vi "Automation Message Loop.vi"(8 "error in (no error)":errorcluster, 9 "Data Queue":refnum<queue>, 10 "Stage Readout Notifier":refnum<notifier>, 11 "Message Queues":T1) -> (0 "error out":errorcluster)   [LabVIEW 2015, in "Automation.lvlib"]
uses:
  Automation.lvlib
  support/Message Queue/All Message Queues.ctl
  support/Message Queue/Message Cluster.ctl
  Automation Configuration.ctl
  Automation State.ctl
  Automation Loop State.ctl
  ZO State.ctl
  ZO Settings.ctl
  Camera/Acquisition Settings.ctl
  Zstack State.ctl
  Zstack Settings.ctl
  Camera/Camera State.ctl
  Camera/Camera Loop State.ctl
  <vilib>/Utility/miscctls.llb/LVMinMaxIncTypeDef.ctl
  Camera/Live View State.ctl
  <vilib>/Utility/error.llb/Error Cluster From Error Code.vi
  <vilib>/ErrorRing/Error Ring.xnode
  support/Message Queue/Message Queue.lvlib
  Camera/Camera.lvlib
  XYZStage/XYZStage.lvlib
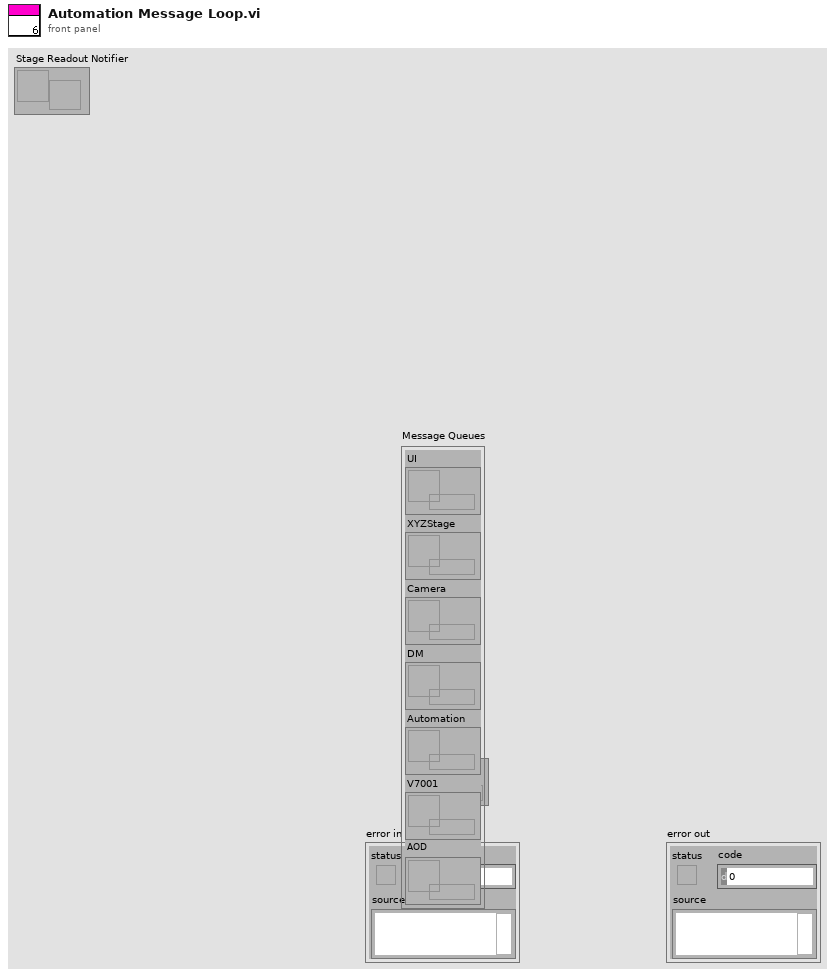
[diagram p1: front panel]
types:
  T1 = typedef "Message Queue.lvlib/All Message Queues.ctl" = cluster{"UI":refnum<queue>, "XYZStage":refnum<queue>, "Camera":refnum<queue>, "DM":refnum<queue>, "Automation":refnum<queue>, "V7001":refnum<queue>, "AOD":refnum<queue>}
  T2 = typedef "Automation.lvlib/Automation State.ctl" = cluster{"Automation State":T3, "Handle out":u32, "ZO State":T4, "Zstack State":T7}
  T3 = typedef "Automation.lvlib/Automation Loop State.ctl" = enum16{"Idle", "Zernike Optimization", "Z Stack"}
  T4 = typedef "Automation.lvlib/ZO State.ctl" = cluster{"ZO Settings":T5, "Zernike Size":i32, "Points per order":i32, "Zernike State":enum16{"Idle", "Waiting for Camera Init.", "Wait for camera frame", "Ready for new mirror config"}, "Zernike Vectors":dbl[][], "Total Frames":i32, "Current Frame":i32}
  T5 = typedef "Automation.lvlib/ZO Settings.ctl" = cluster{"Acquisition Settings":T6, "Shift Amplitude":dbl, "Initial Zernike Vector":dbl[]}
  T6 = typedef "Camera.lvlib/Acquisition Settings.ctl" = cluster{"Save?":bool, "DCIMG Path":path, "Filename":string, "Total Frames":i32, "Sender":enum16{"UI", "Automation"}}
  T7 = typedef "Automation.lvlib/Zstack State.ctl" = cluster{"Zstack Settings":T8, "Zstack State":enum16{"Idle", "Waiting for Camera Init.", "Wait for camera frame", "Ready for new position"}, "Stack Coordinates":dbl[][], "Total Frames":i32, "Current Frame":i32}
  T8 = typedef "Automation.lvlib/Zstack Settings.ctl" = cluster{"Acquisition Settings":T6, "XYZ start":dbl[], "XYZ end":dbl[]}
  T9 = typedef "Automation.lvlib/Automation Configuration.ctl" = cluster{" Index":u32}
  T10 = enum16{"Idle", "Waiting for Camera Init.", "Wait for camera frame", "Ready for new mirror config"}
  T11 = enum16{"Idle", "Waiting for Camera Init.", "Wait for camera frame", "Ready for new position"}
  T12 = typedef "Camera.lvlib/Camera State.ctl" = cluster{"Camera State":T13, "Current Frame":i32, "Handle out":u32, "Camera Details":cluster{"Model":string, "Camera ID":string, "Firmware":string}, "Sub Region":cluster{"H Offset":cluster{"Value":i32, "Limits":T14}, "V Offset":cluster{"Value":i32, "Limits":T14}, "H Size":cluster{"Value":i32, "Limits":T14}, "V Size":cluster{"Value":i32, "Limits":T14}}, "Acquisition Settings":T6, "Live View State":T15}
  T13 = typedef "Camera.lvlib/Camera Loop State.ctl" = enum16{"Idle", "Live View", "Ready", "Acquiring"}
  T14 = typedef "LVMinMaxIncTypeDef.ctl" = cluster{"Minimum":dbl, "Maximum":dbl, "Increment":dbl}
  T15 = typedef "Camera.lvlib/Live View State.ctl" = cluster{"Loop Counter":i32, "Time Of Latest Frame":u32, "Frame Count":u32, "FPS frames":dbl, "FPS Time":u32, "Current FPS":dbl}
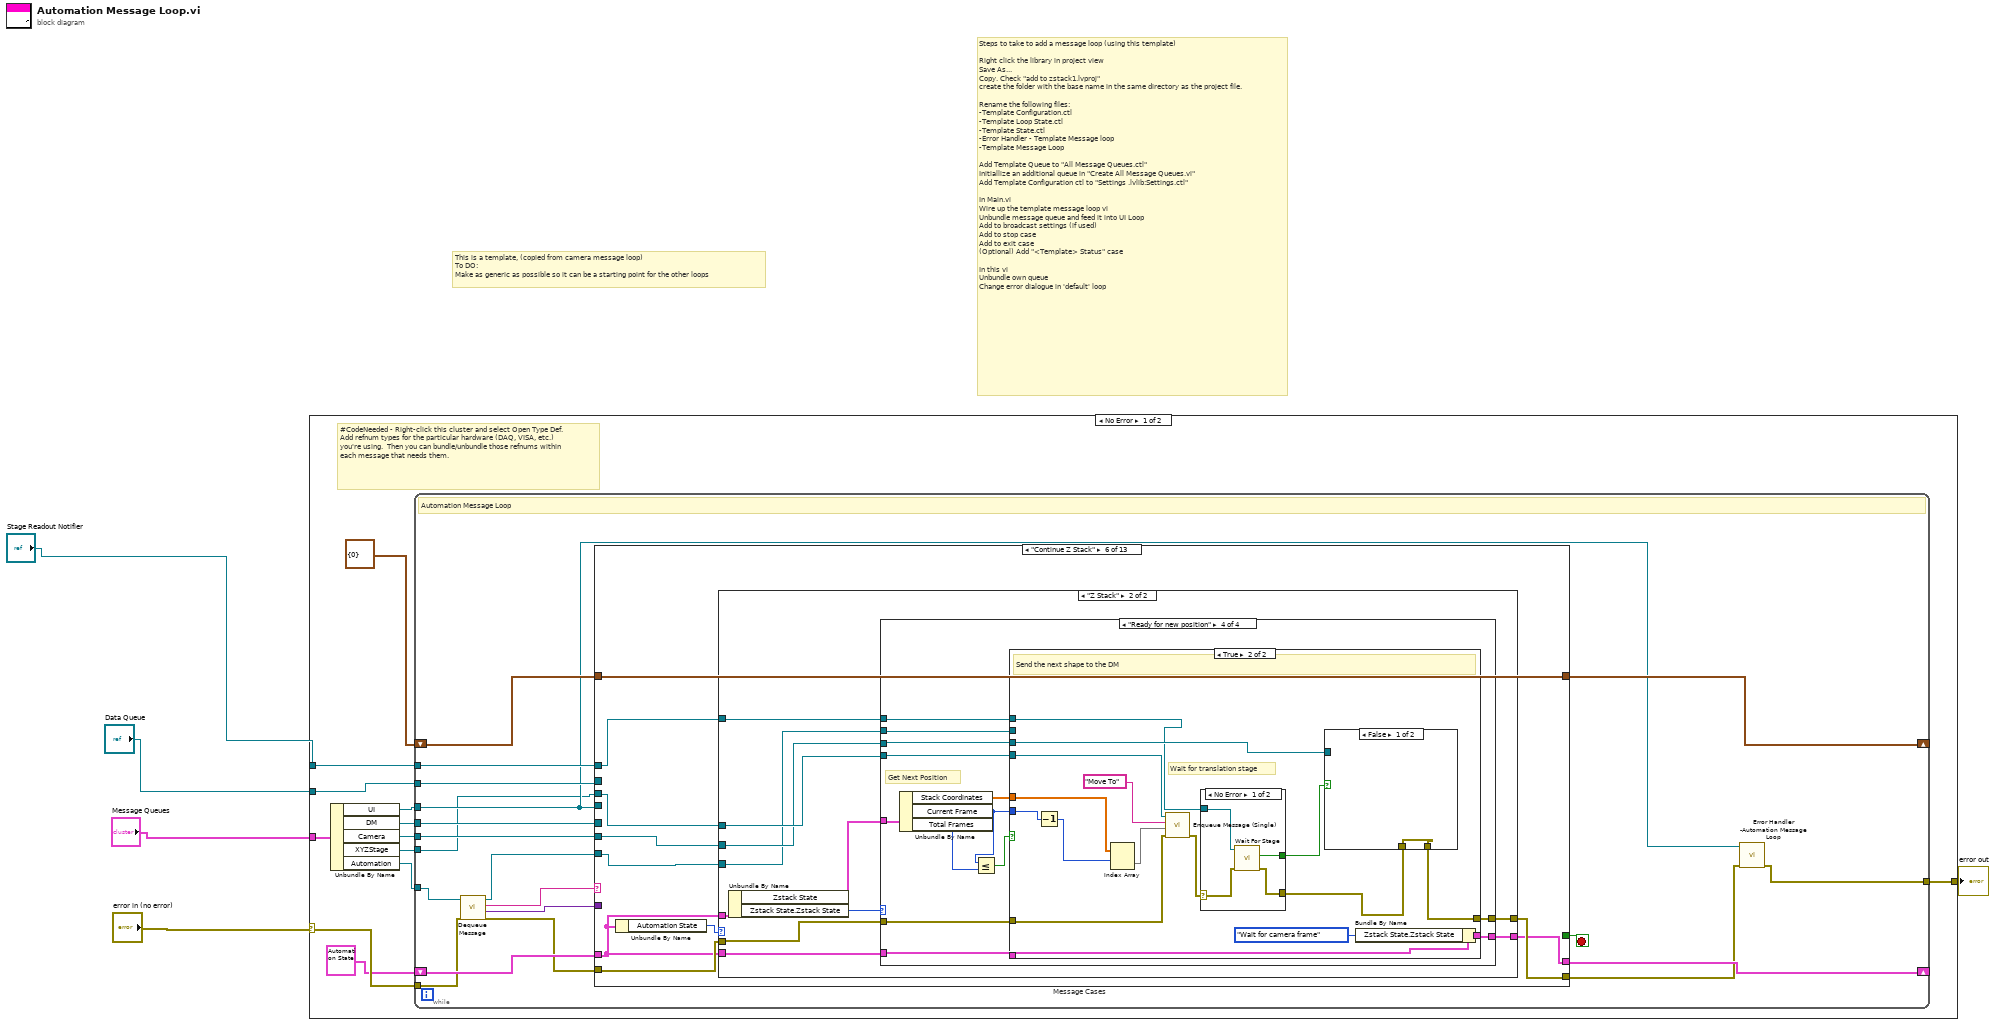
[diagram p0: block diagram]
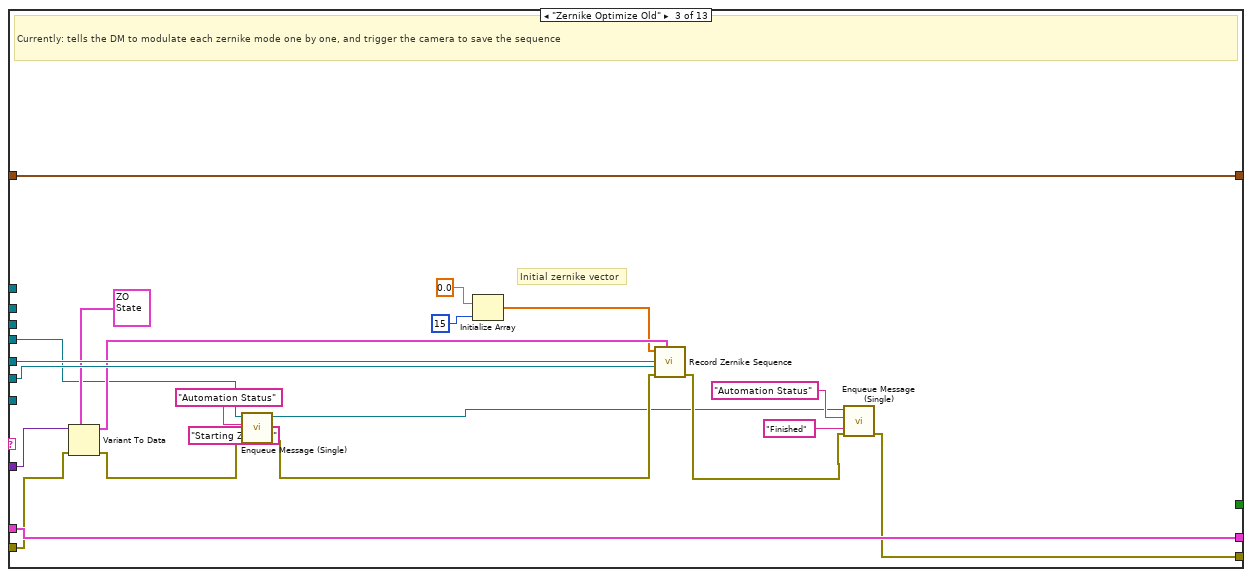
[diagram p4: hidden frame]
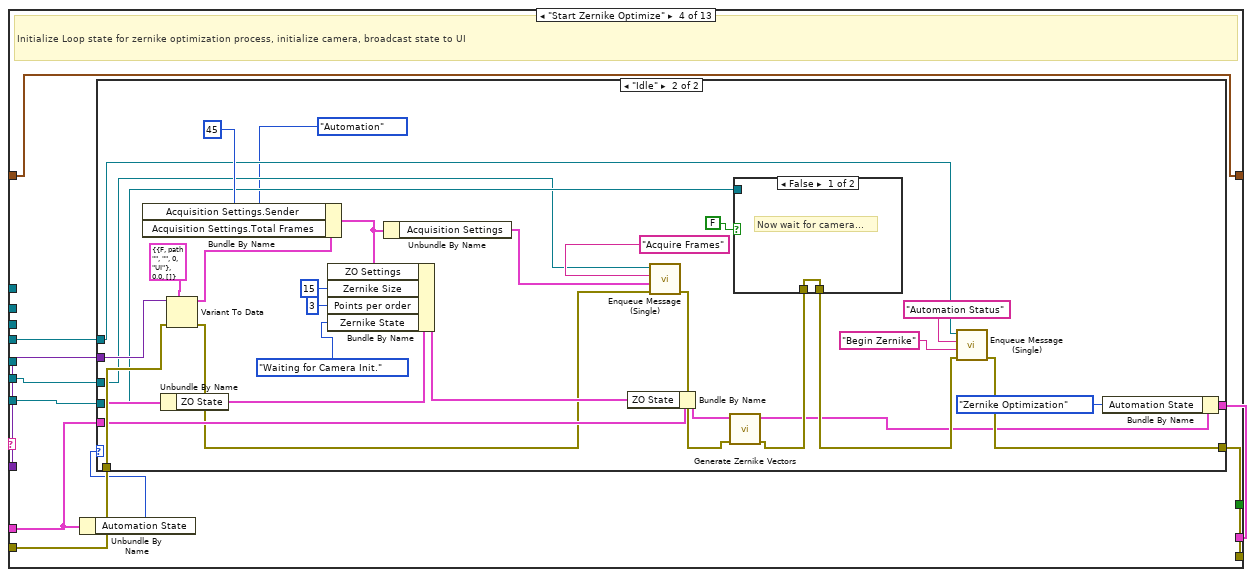
[diagram p5: hidden frame]
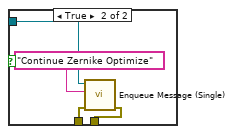
[diagram p7: hidden frame]
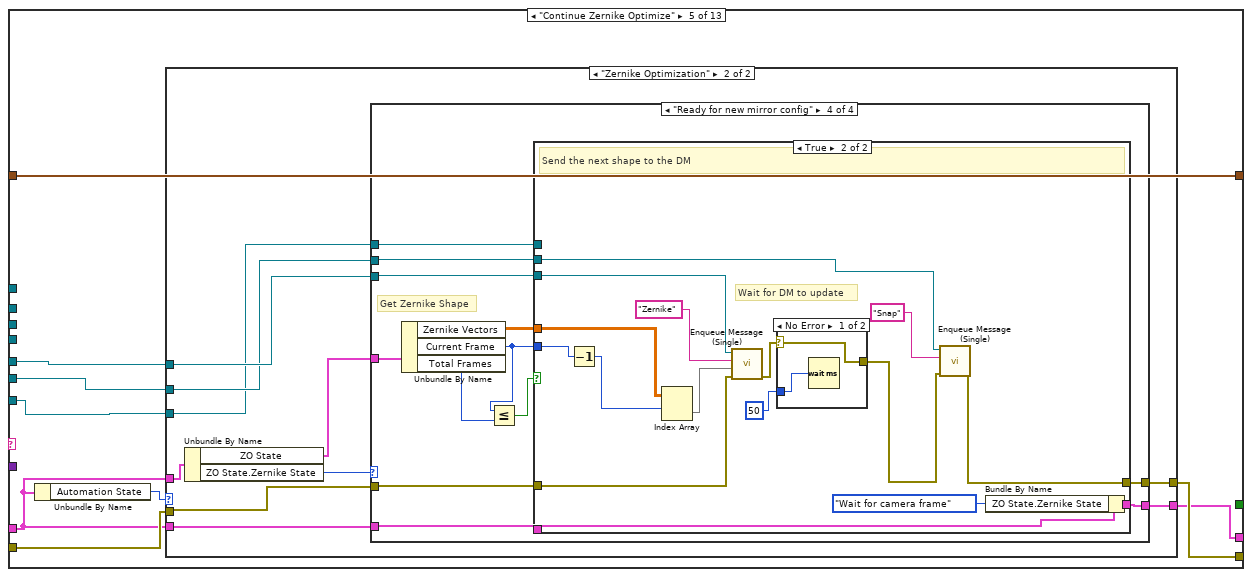
[diagram p8: hidden frame]
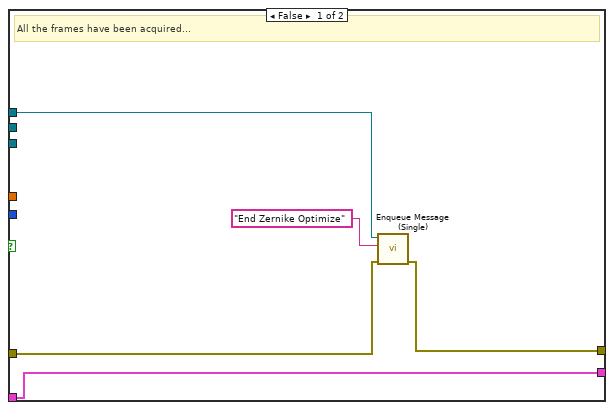
[diagram p13: hidden frame]
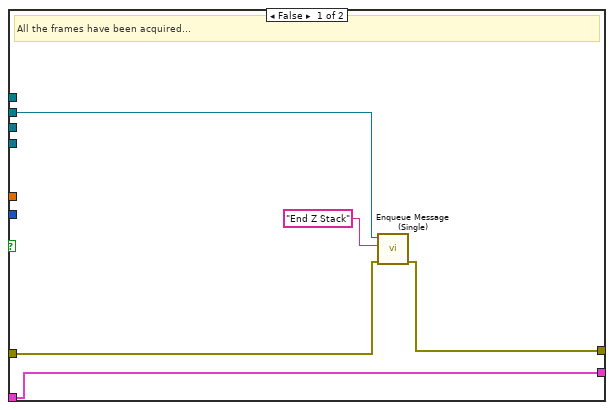
[diagram p19: hidden frame]
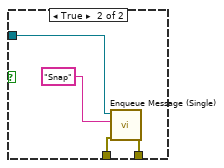
[diagram p20: hidden frame]
diagram:
  # "Steps to take to add a message loop (using this template)\n\nRight click the library in project view\nSave As...\nCopy. Check \"add to zstack1.lvproj\"\ncreate the folder with the base name in the same directory as the project file.\n\nRename the following files:\n-Template Configuration.ctl\n-Template Loop State.ctl\n-Template State.ctl\n-Error Handler - Template Message loop\n-Template Message Loop\n\nAdd Template Queue to \"All Message Queues.ctl\"\nInitiallize an additional queue in \"Create All Message Queues.vi\"\nAdd Template Configuration ctl to \"Settings .lvlib:Settings.ctl\"\n\nIn Main.vi\nWire up the template message loop vi\nUnbundle message queue and feed it into UI Loop\nAdd to broadcast settings (if used)\nAdd to stop case\nAdd to exit case\n(Optional) Add \"<Template> Status\" case\n\nIn this vi\nUnbundle own queue\nChange error dialogue in 'default' loop"
  # "This is a template, (copied from camera message loop)\nTo DO:\nMake as generic as possible so it can be a starting point for the other loops"
  n1 = case shown="No Error" "error in (no error)" {
    selector: "error in (no error)" -> [w15 w469]
    tunnel: "Message Queues" -> [w17 _]
    tunnel: [w16 w469] -> w5
    tunnel: "Stage Readout Notifier" -> [w14 _]
    tunnel: "Data Queue" -> [w13 _]
    frame No Error {
      # "#CodeNeeded - Right-click this cluster and select Open Type Def.  Add refnum types for the particular hardware (DAQ, VISA, etc.) you're using.  Then you can bundle/unbundle those refnums within each message that needs them."
      n2 = Unbundle By Name(w17) -> ("UI"=w10:refnum<queue>, "DM"=w8:refnum<queue>, "Camera"=w7:refnum<queue>, "XYZStage"=w6:refnum<queue>, "Automation"=w9:refnum<queue>)
      n3 = while {
        tunnel: w9 -> [w29]
        shift-right: [w35] -> _
        shift-left: T9 {" Index"=0} ("Hardware Configuration") -> [w36]
        tunnel: w10 -> [w21]
        tunnel: w14 -> [w33]
        tunnel: w13 -> [w32]
        shift-right: [w30] -> _
        shift-left: T2 {"Automation State"=enum."Idle", "Handle out"=0, "ZO State"={"ZO Settings"={"Acquisition Settings"={"Save?"=FALSE, "DCIMG Path"=path "", "Filename"="", "Total Frames"=0, "Sender"=enum."UI"}, "Shift Amplitude"=0.0, "Initial Zernike Vector"=[]}, "Zernike Size"=15, "Points per order"=15, "Zernike State"=enum."Idle", "Zernike Vectors"=[], "Total Frames"=15, "Current Frame"=15}, "Zstack State"={"Zstack Settings"={"Acquisition Settings"={"Save?"=FALSE, "DCIMG Path"=path "", "Filename"="", "Total Frames"=0, "Sender"=enum."UI"}, "XYZ start"=[], "XYZ end"=[]}, "Zstack State"=enum."Idle", "Stack Coordinates"=[], "Total Frames"=15, "Current Frame"=15}} ("Cluster") -> [w31]
        tunnel: w15 -> [w28]
        tunnel: [w23] -> w16
        tunnel: w8 -> [w20]
        tunnel: w7 -> [w19]
        tunnel: w6 -> [w18]
        stop <- w34 stop-if-true
        # "Automation Message Loop"
        n4 = call "Dequeue Message.vi"("error in (no error)"=w28, "Message Queue"=w29) -> ("error out"=w24:errorcluster, "Message Data"=w25:variant, "Message"=w26:string, "dup Message Queue"=w27:refnum<queue>)  [unwired: 6 in]
        n5 = case "Message Cases" shown="\"Continue Z Stack\"" w26 {
          selector: w26 -> [_ _ _ _ _ _ _ _ _ _ _ _ w458]
          tunnel: w27 -> [_ _ _ w68 w111 w176 w255 w285 w306 w331 w448 _ _]
          tunnel: w24 -> [w39 w42 w58 w71 w116 w181 w252 w290 w311 w334 w450 w457 _]
          tunnel: [w39 w42 w44 w70 w115 w180 w251 w289 w310 w329 w452 w455 w459] -> w22
          tunnel: w36 -> [w37 w41 w63 w73 w119 w183 w257 w293 w314 w337 w451 w456 w461]
          tunnel: [w37 w41 w63 w73 w119 w183 w257 w293 w314 w337 w451 w456 w461] -> w35
          tunnel: [_ _ _ _ _ _ _ _ _ _ TRUE _ _] -> w34
          tunnel: w25 -> [_ _ w59 w72 _ _ w248 _ _ w335 _ _ _]
          tunnel: w21 -> [_ _ w51 w69 _ _ w256 w284 w305 _ _ _ _]
          tunnel: w33 -> [_ _ _ _ _ w174 _ _ _ _ _ _ _]
          tunnel: w32 -> [_ _ _ _ _ _ _ _ _ _ _ _ _]
          tunnel: w31 -> [w38 w40 w62 w65 w113 w178 w250 w287 w308 w327 w447 w454 w460]
          tunnel: [w38 w40 w62 w66 w112 w177 w249 w286 w307 w326 w447 w454 w460] -> w30
          tunnel: w20 -> [_ _ w61 _ w117 _ _ w291 w312 _ _ _ _]
          tunnel: w19 -> [_ _ w60 w67 w114 w179 w254 w288 w309 _ _ _ _]
          tunnel: w18 -> [_ _ _ _ _ w175 _ _ _ _ _ _ _]
          frame "Initialize" {
            # "Initialize  - Initialize is currently a no-op.  The hardware initialization takes place in the 'Start' message."
          }
          frame "Stop" {
          }
          frame "Zernike Optimize Old" {
            # "Initial zernike vector"
            # "Currently: tells the DM to modulate each zernike mode one by one, and trigger the camera to save the sequence"
            n6 = Variant To Data(error in=w58, type=T4 {"ZO Settings"={"Acquisition Settings"={"Save?"=FALSE, "DCIMG Path"=path "E:/test2", "Filename"="zernike", "Total Frames"=0, "Sender"=enum."Automation"}, "Shift Amplitude"=0.0, "Initial Zernike Vector"=[]}, "Zernike Size"=15, "Points per order"=15, "Zernike State"=enum."Idle", "Zernike Vectors"=[], "Total Frames"=0, "Current Frame"=15} ("Zernike Optimize Settings"), Variant=w59) -> (data=w56:T4, error out=w50:errorcluster)
            n7 = call "Enqueue Message (Single).vi"("error in (no error)"=w50, "Message Data"="Starting Zernike" ("Message"), "Message"="Automation Status", "Message Queue"=w51) -> ("error out"=w49:errorcluster, "dup Message Queue"=w43:refnum<queue>)  [unwired: 6 in]
            n8 = Initialize Array(0.0 ("element"), 15 ("dimension size")) -> (w55:dbl[])
            n9 = call "Record Zernike Sequence.vi"("Zernike Optimize Settings"=w56, "error in"=w49, "Camera"=w60, "DM"=w61, "Z_0"=w55) -> ("error out"=w45:errorcluster)  [unwired: 6 in]
            n10 = call "Enqueue Message (Single).vi"("error in (no error)"=w45, "Message Data"="Finished" ("Message"), "Message"="Automation Status", "Message Queue"=w43) -> ("error out"=w44:errorcluster)  [unwired: 6 in, 1 out]
          }
          frame "Start Zernike Optimize" {
            # "Initialize Loop state for zernike optimization process, initialize camera, broadcast state to UI"
            n11 = Unbundle By Name(w65) -> ("Automation State"=w64:T3)
            n12 = case shown="\"Idle\"" w64 {
              tunnel: w72 -> [_ w105]
              tunnel: w71 -> [w74 w104]
              tunnel: w65 -> [w75 w103]
              tunnel: [w74 w96] -> w70
              tunnel: w69 -> [_ w95]
              tunnel: w68 -> [_ w94]
              tunnel: w67 -> [_ w91]
              tunnel: [w75 w77] -> w66
              frame Default {
                # "Doing something else!... don't start zernike optimize"
              }
              frame "Idle" {
                n13 = Unbundle By Name(w103) -> ("ZO State"=w99:T4)
                n14 = Variant To Data(error in=w104, type=T5 {"Acquisition Settings"={"Save?"=FALSE, "DCIMG Path"=path "", "Filename"="", "Total Frames"=0, "Sender"=enum."UI"}, "Shift Amplitude"=0.0, "Initial Zernike Vector"=[]} ("ZO Settings"), Variant=w105) -> (data=w100:T5, error out=w88:errorcluster)
                n15 = Bundle By Name(cluster=w100, "Acquisition Settings.Sender"=enum16{"UI", "Automation"}."Automation", "Acquisition Settings.Total Frames"=45) -> (w90:T5)
                n16 = Bundle By Name(cluster=w99, "ZO Settings"=w90, "Zernike Size"=15, "Points per order"=3, "Zernike State"=T10."Waiting for Camera Init.") -> (w98:T4)
                n17 = Unbundle By Name(w90) -> ("Acquisition Settings"=w89:T6)
                n18 = Bundle By Name(cluster=w103, "ZO State"=w98) -> (w82:T2)
                n19 = call "Enqueue Message (Single).vi"("error in (no error)"=w88, "Message Data"=w89, "Message"="Acquire Frames", "Message Queue"=w91) -> ("error out"=w83:errorcluster)  [unwired: 6 in, 1 out]
                n20 = call "Generate Zernike Vectors.vi"("error in (no error)"=w83, "Automation State in"=w82) -> ("error out"=w84:errorcluster, "Automation State Out"=w78:T2)  [unwired: 6 in]
                n21 = case shown="False" FALSE {
                  tunnel: w94 -> [_ w109]
                  tunnel: [w106 w108] -> w93
                  tunnel: w84 -> [w106 w107]
                  frame False {
                    # "Now wait for camera..."
                  }
                  frame True {
                    n22 = call "Enqueue Message (Single).vi"("error in (no error)"=w107, "Message"="Continue Zernike Optimize", "Message Queue"=w109) -> ("error out"=w108:errorcluster)  [unwired: 7 in, 1 out]
                  }
                }
                n23 = call "Enqueue Message (Single).vi"("error in (no error)"=w93, "Message Data"="Begin Zernike" ("Message"), "Message"="Automation Status", "Message Queue"=w95) -> ("error out"=w96:errorcluster)  [unwired: 6 in, 1 out]
                n24 = Bundle By Name(cluster=w78, "Automation State"=Automation_Loop_State."Zernike Optimization") -> (w77:T2)
              }
            }
          }
          frame "Continue Zernike Optimize" {
            n25 = Unbundle By Name(w113) -> ("Automation State"=w118:T3)
            n26 = case shown="\"Zernike Optimization\"" w118 {
              tunnel: w113 -> [_ w131]
              tunnel: w117 -> [_ w128]
              tunnel: w116 -> [w120 w127]
              tunnel: [w120 w126] -> w115
              tunnel: w114 -> [_ w125]
              tunnel: w113 -> [w121 w124]
              tunnel: [w121 w123] -> w112
              tunnel: w111 -> [_ w122]
              frame "Idle", Default {
              }
              frame "Zernike Optimization" {
                n27 = Unbundle By Name(w131) -> ("ZO State"=w129:T4, "ZO State.Zernike State"=w130:T10)
                n28 = case shown="\"Ready for new mirror config\"" w130 {
                  tunnel: w129 -> [_ _ _ w149]
                  tunnel: w128 -> [_ _ _ w147]
                  tunnel: w127 -> [w132 w134 w136 w146]
                  tunnel: [w132 w134 w136 w144] -> w126
                  tunnel: w125 -> [_ _ _ w145]
                  tunnel: w124 -> [w133 w135 w137 w142]
                  tunnel: [w133 w135 w137 w143] -> w123
                  tunnel: w122 -> [_ _ _ w138]
                  frame "Idle", Default {
                  }
                  frame "Waiting for Camera Init." {
                  }
                  frame "Wait for camera frame" {
                  }
                  frame "Ready for new mirror config" {
                    # "Get Zernike Shape"
                    n29 = Unbundle By Name(w149) -> ("Zernike Vectors"=w148:dbl[][], "Current Frame"=w141:i32, "Total Frames"=w140:i32)
                    n30 = Less Or Equal?(x=w141, y=w140) -> (x <= y?=w139:bool)
                    n31 = case shown="True" w139 {
                      tunnel: w148 -> [_ w170]
                      tunnel: w147 -> [_ w165]
                      tunnel: w146 -> [w153 w164]
                      tunnel: w145 -> [_ w163]
                      tunnel: [w152 w160] -> w144
                      tunnel: [w151 w159] -> w143
                      tunnel: w142 -> [w151 w158]
                      tunnel: w141 -> [_ w156]
                      tunnel: w138 -> [w150 _]
                      frame False {
                        # "All the frames have been acquired..."
                        n32 = call "Enqueue Message (Single).vi"("error in (no error)"=w153, "Message"="End Zernike Optimize", "Message Queue"=w150) -> ("error out"=w152:errorcluster)  [unwired: 7 in, 1 out]
                      }
                      frame True {
                        # "Wait for DM to update"
                        # "Send the next shape to the DM"
                        n33 = Decrement(x=w156) -> (x-1=w155:i32)
                        n34 = Index Array(array=w170, index (row)=w155) -> (element=w166:dbl[])  [unwired: 1 in]
                        n35 = call "Enqueue Message (Single).vi"("error in (no error)"=w164, "Message Data"=w166, "Message"="Zernike", "Message Queue"=w165) -> ("error out"=w168:errorcluster)  [unwired: 6 in, 1 out]
                        n36 = case shown="No Error" w168 {
                          selector: w168 -> [w171 w173]
                          tunnel: u32 50 ("milliseconds to wait") -> [w172 _]
                          tunnel: [w171 w173] -> w161
                          frame No Error {
                            n37 = Wait (ms)(milliseconds to wait=w172) -> ()  [unwired: 1 out]
                          }
                          frame Error {
                          }
                        }
                        n38 = call "Enqueue Message (Single).vi"("error in (no error)"=w161, "Message"="Snap", "Message Queue"=w163) -> ("error out"=w160:errorcluster)  [unwired: 7 in, 1 out]
                        n39 = Bundle By Name(cluster=w158, "ZO State.Zernike State"=T10."Wait for camera frame") -> (w159:T2)
                      }
                    }
                  }
                }
              }
            }
          }
          frame "Continue Z Stack" {
            n40 = Unbundle By Name(w178) -> ("Automation State"=w182:T3)
            n41 = case shown="\"Z Stack\"" w182 {
              tunnel: w178 -> [_ w196]
              tunnel: w175 -> [_ w193]
              tunnel: w181 -> [w184 w192]
              tunnel: [w184 w191] -> w180
              tunnel: w179 -> [_ w190]
              tunnel: w178 -> [w185 w189]
              tunnel: [w185 w188] -> w177
              tunnel: w176 -> [_ w187]
              tunnel: w174 -> [_ w186]
              frame "Idle", Default {
              }
              frame "Z Stack" {
                n42 = Unbundle By Name(w196) -> ("Zstack State"=w194:T7, "Zstack State.Zstack State"=w195:T11)
                n43 = case shown="\"Ready for new position\"" w195 {
                  tunnel: w194 -> [_ _ _ w215]
                  tunnel: w193 -> [_ _ _ w213]
                  tunnel: w192 -> [w197 w199 w201 w212]
                  tunnel: [w197 w199 w201 w210] -> w191
                  tunnel: w190 -> [_ _ _ w211]
                  tunnel: w189 -> [w198 w200 w202 w208]
                  tunnel: [w198 w200 w202 w209] -> w188
                  tunnel: w187 -> [_ _ _ w204]
                  tunnel: w186 -> [_ _ _ w203]
                  frame "Idle", Default {
                  }
                  frame "Waiting for Camera Init." {
                  }
                  frame "Wait for camera frame" {
                  }
                  frame "Ready for new position" {
                    # "Get Next Position"
                    n44 = Unbundle By Name(w215) -> ("Stack Coordinates"=w214:dbl[][], "Current Frame"=w207:i32, "Total Frames"=w206:i32)
                    n45 = Less Or Equal?(x=w207, y=w206) -> (x <= y?=w205:bool)
                    n46 = case shown="True" w205 {
                      tunnel: w214 -> [_ w236]
                      tunnel: w213 -> [_ w232]
                      tunnel: w212 -> [w219 w231]
                      tunnel: w211 -> [_ w230]
                      tunnel: [w218 w228] -> w210
                      tunnel: [w217 w227] -> w209
                      tunnel: w208 -> [w217 w226]
                      tunnel: w207 -> [_ w225]
                      tunnel: w204 -> [w216 _]
                      tunnel: w203 -> [_ w221]
                      frame False {
                        # "All the frames have been acquired..."
                        n47 = call "Enqueue Message (Single).vi"("error in (no error)"=w219, "Message"="End Z Stack", "Message Queue"=w216) -> ("error out"=w218:errorcluster)  [unwired: 7 in, 1 out]
                      }
                      frame True {
                        # "Wait for translation stage"
                        # "Send the next shape to the DM"
                        n48 = Decrement(x=w225) -> (x-1=w224:i32)
                        n49 = Index Array(array=w236, index (row)=w224) -> (element=w233:dbl[])  [unwired: 1 in]
                        n50 = call "Enqueue Message (Single).vi"("error in (no error)"=w231, "Message Data"=w233, "Message"="Move To", "Message Queue"=w232) -> ("error out"=w234:errorcluster)  [unwired: 6 in, 1 out]
                        n51 = case shown="No Error" w234 {
                          selector: w234 -> [w245 w247]
                          tunnel: [w244 w247] -> w229
                          tunnel: [w243 FALSE ("In Position")] -> w222
                          tunnel: w221 -> [w242 _]
                          frame No Error {
                            n52 = call "Wait For Stage.vi"("error in (no error)"=w245, "Stage Readout Notifier"=w242) -> ("error out"=w244:errorcluster, "In Position"=w243:bool)  [unwired: 8 in]
                          }
                          frame Error {
                          }
                        }
                        n53 = case shown="False" w222 {
                          tunnel: w230 -> [_ w241]
                          tunnel: w229 -> [w237 w239]
                          tunnel: [w237 w238] -> w228
                          frame False {
                          }
                          frame True {
                            n54 = call "Enqueue Message (Single).vi"("error in (no error)"=w239, "Message"="Snap", "Message Queue"=w241) -> ("error out"=w238:errorcluster)  [unwired: 7 in, 1 out]
                          }
                        }
                        n55 = Bundle By Name(cluster=w226, "Zstack State.Zstack State"=T11."Wait for camera frame") -> (w227:T2)
                      }
                    }
                  }
                }
              }
            }
          }
          frame "Start Z Stack" {
            n56 = Unbundle By Name(w250) -> ("Automation State"=w253:T3)
            n57 = case shown="Default" w253 {
              tunnel: w248 -> [_ w278]
              tunnel: w252 -> [w258 w277]
              tunnel: w250 -> [w259 w265]
              tunnel: [w258 w275] -> w251
              tunnel: w256 -> [_ w274]
              tunnel: w255 -> [_ w273]
              tunnel: w254 -> [_ w270]
              tunnel: [w259 w261] -> w249
              frame Default {
                # "Doing something else!... don't start zernike optimize"
              }
              frame "Idle" {
                # "initialize camera"
                n58 = Variant To Data(error in=w277, type=T8 {"Acquisition Settings"={"Save?"=FALSE, "DCIMG Path"=path "", "Filename"="", "Total Frames"=0, "Sender"=enum."UI"}, "XYZ start"=[], "XYZ end"=[]} ("Zstack Settings"), Variant=w278) -> (data=w264:T8, error out=w263:errorcluster)
                n59 = call "Initialize Z Stack.vi"("error in (no error)"=w263, "Zstack Settings in"=w264, "Automation State in"=w265) -> ("error out"=w262:errorcluster, "Automation State Out"=w261:T2)  [unwired: 5 in]
                n60 = Unbundle By Name(w261) -> ("Zstack State.Zstack Settings.Acquisition Settings"=w260:T6)
                n61 = call "Enqueue Message (Single).vi"("error in (no error)"=w262, "Message Data"=w260, "Message"="Acquire Frames", "Message Queue"=w270) -> ("error out"=w266:errorcluster)  [unwired: 6 in, 1 out]
                n62 = case shown="False" FALSE {
                  tunnel: w273 -> [_ w282]
                  tunnel: [w279 w281] -> w272
                  tunnel: w266 -> [w279 w280]
                  frame False {
                    # "Now wait for camera..."
                  }
                  frame True {
                    n63 = call "Enqueue Message (Single).vi"("error in (no error)"=w280, "Message"="Continue Zernike Optimize", "Message Queue"=w282) -> ("error out"=w281:errorcluster)  [unwired: 7 in, 1 out]
                  }
                }
                n64 = call "Enqueue Message (Single).vi"("error in (no error)"=w272, "Message Data"="Begin Z Stack" ("Message"), "Message"="Automation Status", "Message Queue"=w274) -> ("error out"=w275:errorcluster)  [unwired: 6 in, 1 out]
              }
            }
          }
          frame "End Zernike Optimize" {
            # "Clear settings and set loop state to idle..."
            n65 = Unbundle By Name(w287) -> ("Automation State"=w292:T3)
            n66 = case shown="\"Zernike Optimization\"" w292 {
              tunnel: w287 -> [_ _]
              tunnel: w291 -> [_ _]
              tunnel: w290 -> [w294 w297]
              tunnel: [w294 w296] -> w289
              tunnel: w288 -> [_ _]
              tunnel: w287 -> [w295 w301]
              tunnel: [w295 w300] -> w286
              tunnel: w285 -> [_ _]
              tunnel: w284 -> [_ w304]
              frame "Idle", Default {
              }
              frame "Zernike Optimization" {
                n67 = call "Enqueue Message (Single).vi"("error in (no error)"=w297, "Message Data"="Zernike Measurement Complete" ("Message"), "Message"="Automation Status", "Message Queue"=w304) -> ("error out"=w296:errorcluster)  [unwired: 6 in, 1 out]
                n68 = Bundle By Name(cluster=w301, "Automation State"=Automation_Loop_State."Idle", "ZO State"=T4 {"ZO Settings"={"Acquisition Settings"={"Save?"=FALSE, "DCIMG Path"=path "", "Filename"="", "Total Frames"=0, "Sender"=enum."UI"}, "Shift Amplitude"=0.0, "Initial Zernike Vector"=[]}, "Zernike Size"=15, "Points per order"=3, "Zernike State"=enum."Ready for new mirror config", "Zernike Vectors"=[], "Total Frames"=1, "Current Frame"=1}) -> (w300:T2)
              }
            }
          }
          frame "End Z Stack" {
            # "Clear settings and set loop state to idle..."
            n69 = Unbundle By Name(w308) -> ("Automation State"=w313:T3)
            n70 = case shown="\"Z Stack\"" w313 {
              tunnel: w308 -> [_ _]
              tunnel: w312 -> [_ _]
              tunnel: w311 -> [w315 w319]
              tunnel: [w315 w318] -> w310
              tunnel: w309 -> [_ _]
              tunnel: w308 -> [w316 w322]
              tunnel: [w316 w321] -> w307
              tunnel: w306 -> [_ _]
              tunnel: w305 -> [_ w325]
              frame "Idle", Default {
              }
              frame "Z Stack" {
                n71 = call "Enqueue Message (Single).vi"("error in (no error)"=w319, "Message Data"="ZStack Complete" ("Message"), "Message"="Automation Status", "Message Queue"=w325) -> ("error out"=w318:errorcluster)  [unwired: 6 in, 1 out]
                n72 = Bundle By Name(cluster=w322, "Automation State"=Automation_Loop_State."Idle", "Zstack State"=T7 {"Zstack Settings"={"Acquisition Settings"={"Save?"=FALSE, "DCIMG Path"=path "", "Filename"="", "Total Frames"=0, "Sender"=enum."UI"}, "XYZ start"=[], "XYZ end"=[]}, "Zstack State"=enum."Idle", "Stack Coordinates"=[], "Total Frames"=15, "Current Frame"=15}) -> (w321:T2)
              }
            }
          }
          frame "Camera Status" {
            # "If the automator is waiting for the camera to do something, the command from the camera happens here..."
            n73 = Variant To Data(error in=w334, type=T12 {"Camera State"=enum."Idle", "Current Frame"=0, "Handle out"=0, "Camera Details"={"Model"="", "Camera ID"="", "Firmware"=""}, "Sub Region"={"H Offset"={"Value"=0, "Limits"={"Minimum"=0.0, "Maximum"=0.0, "Increment"=0.0}}, "V Offset"={"Value"=0, "Limits"={"Minimum"=0.0, "Maximum"=0.0, "Increment"=0.0}}, "H Size"={"Value"=0, "Limits"={"Minimum"=0.0, "Maximum"=0.0, "Increment"=0.0}}, "V Size"={"Value"=0, "Limits"={"Minimum"=0.0, "Maximum"=0.0, "Increment"=0.0}}}, "Acquisition Settings"={"Save?"=FALSE, "DCIMG Path"=path "", "Filename"="", "Total Frames"=0, "Sender"=enum."UI"}, "Live View State"={"Loop Counter"=0, "Time Of Latest Frame"=0, "Frame Count"=0, "FPS frames"=0.0, "FPS Time"=0, "Current FPS"=0.0}} ("Cluster"), Variant=w335) -> (data=w332:T12, error out=w330:errorcluster)
            n74 = Unbundle By Name(w327) -> ("Automation State"=w333:T3)
            n75 = case shown="\"Z Stack\"" w333 {
              tunnel: w327 -> [w338 w341 w395]
              tunnel: w332 -> [_ w339 w393]
              tunnel: w331 -> [_ w345 w399]
              tunnel: [_ w343 w397] -> w328
              tunnel: [w338 w342 w396] -> w326
              frame "Idle", Default {
              }
              frame "Zernike Optimization" {
                n76 = Unbundle By Name(w341) -> ("ZO State"=w344:T4)
                n77 = Unbundle By Name(w344) -> ("Zernike State"=w346:T10)
                n78 = case shown="\"Waiting for Camera Init.\"" w346 {
                  tunnel: w339 -> [_ w353 w368 _]
                  tunnel: w345 -> [_ w351 w366 _]
                  tunnel: w344 -> [w347 w350 w365 w392]
                  tunnel: [_ w349 w364 _] -> w343
                  tunnel: [w347 w348 w363 w392] -> w340
                  frame "Idle", Default {
                  }
                  frame "Waiting for Camera Init." {
                    n79 = Unbundle By Name(w353) -> ("Camera State"=w352:T13)
                    n80 = case shown="\"Acquiring\"" w352 {
                      tunnel: w351 -> [_ w361]
                      tunnel: w350 -> [w354 w359]
                      tunnel: [_ w357] -> w349
                      tunnel: [w354 w356] -> w348
                      frame "Idle", Default {
                      }
                      frame "Acquiring" {
                        # "Camera has initialized"
                        n81 = call "Enqueue Message (Single).vi"("Message"="Continue Zernike Optimize", "Message Queue"=w361) -> ("error out"=w357:errorcluster)  [unwired: 8 in, 1 out]
                        n82 = Bundle By Name(cluster=w359, "Current Frame"=1, "Zernike State"=T10."Ready for new mirror config") -> (w356:T4)
                      }
                    }
                  }
                  frame "Wait for camera frame" {
                    n83 = Unbundle By Name(w368) -> ("Current Frame"=w362:i32, "Camera State"=w367:T13)
                    n84 = case shown="\"Acquiring\"" w367 {
                      tunnel: w366 -> [_ w376]
                      tunnel: w365 -> [w369 w373]
                      tunnel: [_ w375] -> w364
                      tunnel: [w369 w374] -> w363
                      tunnel: w362 -> [_ w372]
                      frame "Idle", Default {
                      }
                      frame "Acquiring" {
                        # "Camera has initialized"
                        n85 = Unbundle By Name(w373) -> ("Current Frame"=w370:i32)
                        n86 = Equal?(x=w372, y=w370) -> (x = y?=w371:bool)
                        n87 = case shown="True" w371 {
                          tunnel: w376 -> [_ w391]
                          tunnel: [w377 w388] -> w375
                          tunnel: [w378 w387] -> w374
                          tunnel: w373 -> [w378 w386]
                          tunnel: w370 -> [_ w385]
                          frame False {
                            n88 = xnode "Error Ring"() -> ("error out"=w377:errorcluster)
                          }
                          frame True {
                            # "Frame is complete... increment frame"
                            n89 = Increment(x=w385) -> (x+1=w384:i32)
                            n90 = call "Enqueue Message (Single).vi"("Message"="Continue Zernike Optimize", "Message Queue"=w391) -> ("error out"=w388:errorcluster)  [unwired: 8 in, 1 out]
                            n91 = Bundle By Name(cluster=w386, "Current Frame"=w384, "Zernike State"=T10."Ready for new mirror config") -> (w387:T4)
                          }
                        }
                      }
                    }
                  }
                  frame "Ready for new mirror config" {
                  }
                }
                n92 = Bundle By Name(cluster=w341, "ZO State"=w340) -> (w342:T2)
              }
              frame "Z Stack" {
                n93 = Unbundle By Name(w395) -> ("Zstack State"=w398:T7)
                n94 = Unbundle By Name(w398) -> ("Zstack State"=w400:T11)
                n95 = case shown="\"Wait for camera frame\"" w400 {
                  tunnel: w393 -> [_ w407 w422 _]
                  tunnel: w399 -> [_ w405 w420 _]
                  tunnel: w398 -> [w401 w404 w419 w446]
                  tunnel: [_ w403 w418 _] -> w397
                  tunnel: [w401 w402 w417 w446] -> w394
                  frame "Idle", Default {
                  }
                  frame "Waiting for Camera Init." {
                    n96 = Unbundle By Name(w407) -> ("Camera State"=w406:T13)
                    n97 = case shown="\"Acquiring\"" w406 {
                      tunnel: w405 -> [_ w415]
                      tunnel: w404 -> [w408 w413]
                      tunnel: [_ w412] -> w403
                      tunnel: [w408 w411] -> w402
                      frame "Idle", Default {
                      }
                      frame "Acquiring" {
                        # "Camera has initialized"
                        n98 = call "Enqueue Message (Single).vi"("Message"="Continue Z Stack", "Message Queue"=w415) -> ("error out"=w412:errorcluster)  [unwired: 8 in, 1 out]
                        n99 = Bundle By Name(cluster=w413, "Current Frame"=1, "Zstack State"=T11."Ready for new position") -> (w411:T7)
                      }
                    }
                  }
                  frame "Wait for camera frame" {
                    n100 = Unbundle By Name(w422) -> ("Current Frame"=w416:i32, "Camera State"=w421:T13)
                    n101 = case shown="\"Acquiring\"" w421 {
                      tunnel: w420 -> [_ w430]
                      tunnel: w419 -> [w423 w427]
                      tunnel: [_ w429] -> w418
                      tunnel: [w423 w428] -> w417
                      tunnel: w416 -> [_ w426]
                      frame "Idle", Default {
                      }
                      frame "Acquiring" {
                        # "Camera has initialized"
                        n102 = Unbundle By Name(w427) -> ("Current Frame"=w424:i32)
                        n103 = Equal?(x=w426, y=w424) -> (x = y?=w425:bool)
                        n104 = case shown="True" w425 {
                          tunnel: w430 -> [_ w445]
                          tunnel: [w431 w442] -> w429
                          tunnel: [w432 w441] -> w428
                          tunnel: w427 -> [w432 w440]
                          tunnel: w424 -> [_ w439]
                          frame False {
                            n105 = xnode "Error Ring"() -> ("error out"=w431:errorcluster)
                          }
                          frame True {
                            # "Frame is complete... increment frame"
                            n106 = Increment(x=w439) -> (x+1=w438:i32)
                            n107 = call "Enqueue Message (Single).vi"("Message"="Continue Z Stack", "Message Queue"=w445) -> ("error out"=w442:errorcluster)  [unwired: 8 in, 1 out]
                            n108 = Bundle By Name(cluster=w440, "Current Frame"=w438, "Zstack State"=T11."Ready for new position") -> (w441:T7)
                          }
                        }
                      }
                    }
                  }
                  frame "Ready for new position" {
                  }
                }
                n109 = Bundle By Name(cluster=w395, "Zstack State"=w394) -> (w396:T2)
              }
            }
            n110 = Merge Errors(w328, w330) -> (w329:errorcluster)
          }
          frame "Exit" {
            # "Release the Acquisition queue reference"
            # "Stop the VI"
            # "Exit - Send the Exit message to the UI Message Handler."
            n111 = Release Queue(queue=w448, error in (no error)=w450) -> (error out=w449:errorcluster)  [unwired: 1 in, 2 out]
            n112 = Merge Errors(w449) -> (w452:errorcluster)
          }
          frame "---Copy This Frame---" {
            # "Duplicate this frame when creating new messages.  Change this comment in the duplicated frame to describe this message."
            n113 = Merge Errors(w457) -> (w455:errorcluster)
          }
          frame Default {
            # "'Default' case only runs if there is a message that isn't defined in any of the other cases.  Output a programming error."
            n114 = xnode "Error Ring"("parameter 0"=w458) -> ("error out"=w459:errorcluster)
          }
        }
        n115 = call "Error Handler -Automation Message Loop.vi"("error in (no error)"=w22, "Message Queue"=w21) -> ("dup error in"=w23:errorcluster)  [unwired: 8 in, 1 out]
      }
    }
    frame Error {
    }
  }
  "error out" <- w5
